vi "background acquisition.vi"(7 "File path":path, 8 "Error IN":errorcluster, 9 "Ydim":u32, 10 "Xdim":u32, 11 "Camera Handle":u32) -> (0 "Error OUT":errorcluster, 3 "BackIsOK":bool)   [LabVIEW 2020]
panel:
  in  "SITKFULLDISPLAYLib.SITKFullDisplay":refnum<k7>(container)
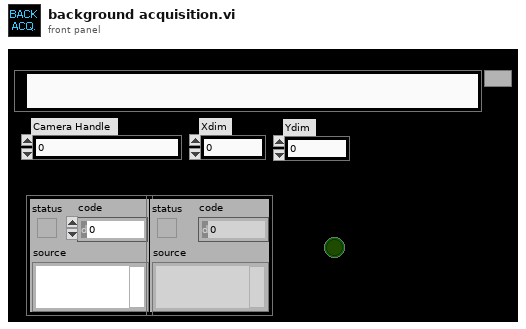
[diagram p1: front panel]
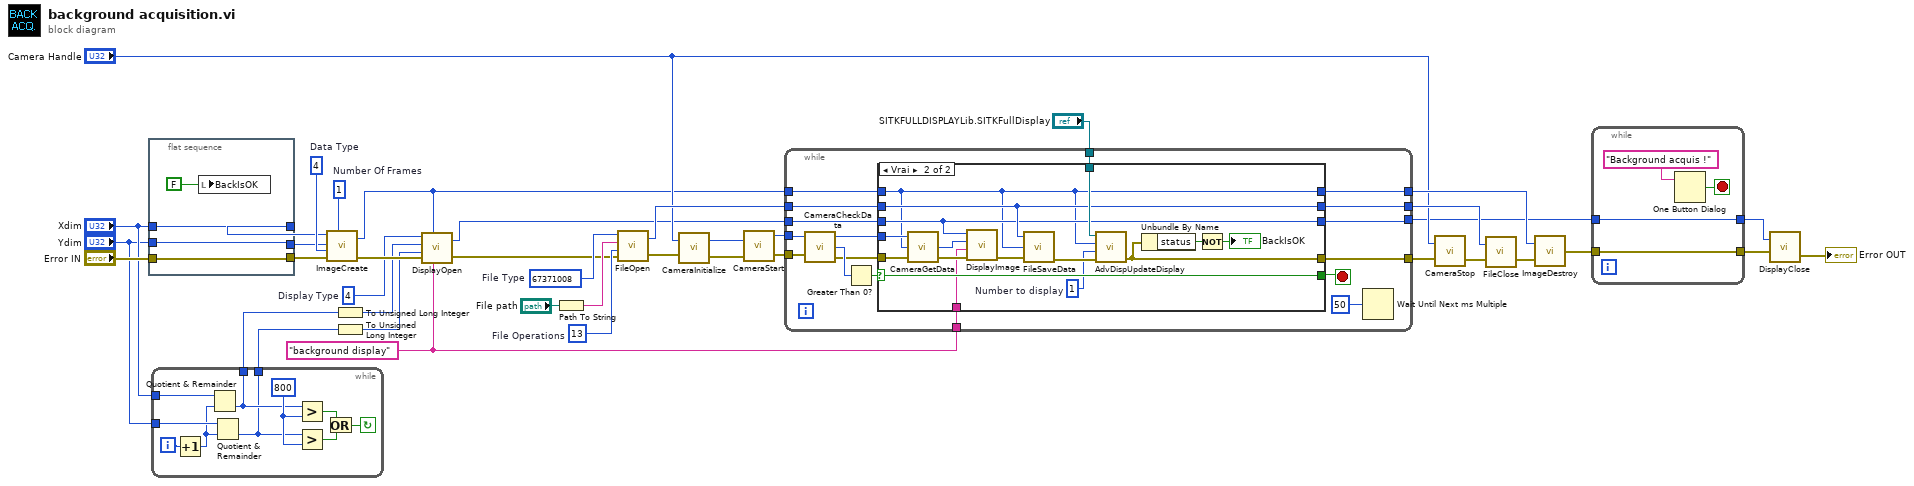
[diagram p0: block diagram]
diagram:
  w10 = u32 4  # Display Type
  w8 = "background display" ("Display Title")
  w35 = 13  # File Operations
  w37 = 67371008  # File Type
  w38 = u32 4  # Data Type
  w39 = u32 1  # Number Of Frames
  n1 = flat-sequence {
    tunnel: [w44] -> w22
    tunnel: "Xdim" -> [w44]
    tunnel: [w43] -> w21
    tunnel: "Ydim" -> [w43]
    tunnel: [w42] -> w19
    tunnel: "Error IN" -> [w42]
    frame #0 {
      n2 = local write "BackIsOK"(FALSE ("BackIsOK")) -> ()
    }
  }
  n3 = while {
    tunnel: "Xdim" -> [w53]
    tunnel: "Ydim" -> [w52]
    tunnel: [w47] -> w14
    tunnel: [w46] -> w13
    i -> [w51]
    stop <- w48 continue-if-true
    w54 = 800
    n4 = Increment(x=w51) -> (x+1=w45:i32)
    n5 = Quotient & Remainder(x=w53, y=w45) -> (floor(x/y)=w47:u32)  [unwired: 1 out]
    n6 = Quotient & Remainder(x=w52, y=w45) -> (floor(x/y)=w46:u32)  [unwired: 1 out]
    n7 = Greater?(x=w47, y=w54) -> (0:w50:bool)
    n8 = Greater?(x=w46, y=w54) -> (0:w49:bool)
    n9 = Or(x=w50, y=w49) -> (x .or. y?=w48:bool)
  }
  n10 = call <userlib>:"ImageCreate.vi"("X dimension"=w22, "Y dimension"=w21, "Data Type"=w38, "error in"=w19, "Number Of Frames"=w39) -> ("Image Handle"=w9:u32, "error out"=w18:errorcluster)
  n11 = To Unsigned Long Integer(number=w14) -> (unsigned 32bit integer=w12:u32)
  n12 = To Unsigned Long Integer(number=w13) -> (unsigned 32bit integer=w11:u32)
  n13 = call <userlib>:"DisplayOpen.vi"("Display Title"=w8, "Image Handle"=w9, "error in"=w18, "Display Height"=w11, "Display Width"=w12, "Display Type"=w10) -> ("error out"=w17:errorcluster, "Display Handle"=w7:u32)
  n14 = Path To String(path="File path") -> (string=w36:string)
  n15 = call <userlib>:"FileOpen.vi"("error in"=w17, "File Operations"=w35, "FileName"=w36, "File Type"=w37) -> ("error out"=w26:errorcluster, "File Handle"=w32:u32)
  n16 = call <userlib>:"CameraInitialize.vi"("error in"=w26, "Camera Handle"="Camera Handle") -> ("error out"=w25:errorcluster, "Camera Handle"=w24:u32)
  n17 = call <userlib>:"CameraStart.vi"("error in"=w25, "Camera Handle"=w24) -> ("error out"=w34:errorcluster, "Camera Handle"=w33:u32)
  n18 = while {
    tunnel: w34 -> [w70]
    tunnel: w33 -> [w69]
    tunnel: [w64] -> w30
    tunnel: w9 -> [w62]
    tunnel: w32 -> [w61]
    tunnel: "SITKFULLDISPLAYLib.SITKFullDisplay" -> [w60]
    tunnel: [w59] -> w28
    tunnel: [w58] -> w27
    tunnel: w8 -> [w57]
    tunnel: w7 -> [w56]
    tunnel: [w55] -> w2
    stop <- w65 stop-if-true
    n19 = call <userlib>:"CameraCheckData.vi"("Camera Handle"=w69, "error in"=w70) -> ("Camera Handle"=w67:u32, "Number Of Frames Available"=w71:i32, "error out"=w66:errorcluster)
    n20 = Greater Than 0?(x=w71) -> (x > 0?=w68:bool)
    n21 = case shown="Vrai" w68 {
      selector: w68 -> [w75 w90]
      tunnel: w67 -> [_ w92]
      tunnel: w66 -> [w76 w91]
      tunnel: [w75 w90] -> w65
      tunnel: [w76 w85] -> w64
      tunnel: w62 -> [w74 w77]
      tunnel: w61 -> [w73 w86]
      tunnel: w60 -> [_ w87]
      tunnel: [w73 w86] -> w59
      tunnel: [w74 w77] -> w58
      tunnel: w57 -> [_ w79]
      tunnel: w56 -> [w72 w78]
      tunnel: [w72 w78] -> w55
      frame False {
      }
      frame True {
        w88 = 1  # Number to display
        n22 = call <userlib>:"CameraGetData.vi"("error in"=w91, "Image/Data Handle"=w77, "Camera Handle"=w92) -> ("error out"=w82:errorcluster, "Image/Data Handle"=w80:u32)  [unwired: 1 out]
        n23 = call <userlib>:"DisplayImage.vi"("error in"=w82, "Title"=w79, "Image Handle"=w80, "Display Handle"=w78) -> ("error out"=w81:errorcluster)  [unwired: 1 out]
        n24 = call <userlib>:"FileSaveData.vi"("error in"=w81, "Image Handle"=w77, "File Handle"=w86) -> ("error out"=w89:errorcluster)  [unwired: 1 out]
        n25 = call <userlib>:"AdvDispUpdateDisplay.vi"("error in (no error)"=w89, "Frame Number To Display"=w88, "Image Handle"=w77, "SITKFULLDISPLAYLib.SITKFullDisplay"=w87) -> ("error out"=w85:errorcluster)  [unwired: 1 out]
        n26 = Unbundle By Name(w85) -> ("status"=w84:bool)
        n27 = Not(x=w84) -> (.not. x?=→"BackIsOK":bool)
      }
    }
    n28 = Wait Until Next ms Multiple(millisecond multiple=u32 50) -> ()  [unwired: 1 out]
  }
  n29 = call <userlib>:"CameraStop.vi"("error in"=w30, "Camera Handle"="Camera Handle") -> ("error out"=w6:errorcluster)  [unwired: 1 out]
  n30 = call <userlib>:"FileClose.vi"("error in"=w6, "File Handle"=w28) -> ("error out"=w29:errorcluster)
  n31 = call <userlib>:"ImageDestroy.vi"("error in"=w29, "Data handle"=w27) -> ("error out"=w4:errorcluster)
  n32 = while {
    tunnel: w4 -> [w96]
    tunnel: [w96] -> w3
    tunnel: w2 -> [w95]
    tunnel: [w95] -> w1
    stop <- w94 stop-if-true
    n33 = One Button Dialog(message="Background acquis !") -> (true=w94:bool)  [unwired: 1 in]
  }
  n34 = call <userlib>:"DisplayClose.vi"("error in"=w3, "Display Handle"=w1) -> ("error out"=→"Error OUT":errorcluster)
